vi "Cmd_G_OK.vi"(0 "Residence time":i32=100, 1 "PortNumber":i32=7, 2 "Command String":string) -> (3 "Received String1":string, 4 "Received String2":string, 5 "Received String3":string, 6 "OK Done":bool)   [LabVIEW 2015]
panel:
  # "Port Number 0=COM1"
  # "Send 'Command String', receive 'OK', send 'G Command' and receive 'OK'."
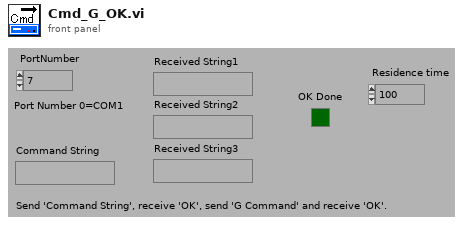
[diagram p1: front panel]
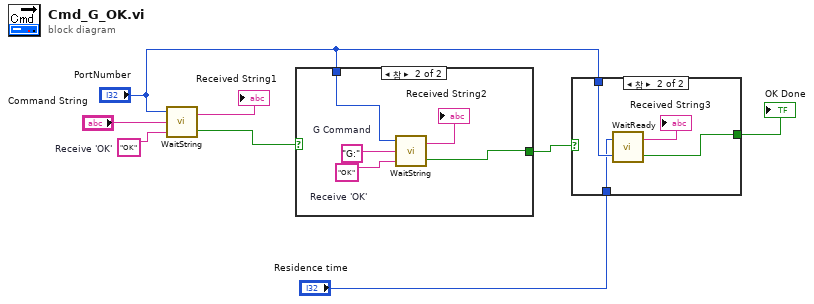
[diagram p0: block diagram]
diagram:
  w4 = "OK"  # Receive 'OK'
  n1 = call "WaitString.vi"("String to Receive"=w4, "String to Send"="Command String", "PortNumber"="PortNumber") -> ("OK Done"=w2:bool, "String Received"=→"Received String1":string)
  n2 = case shown="참" w2 {
    selector: w2 -> [w9 _]
    tunnel: "PortNumber" -> [_ w14]
    tunnel: [w9 w10] -> w7
    frame False {
    }
    frame True {
      w12 = "OK"  # Receive 'OK'
      w13 = "G:"  # G Command
      n3 = call "WaitString.vi"("String to Receive"=w12, "String to Send"=w13, "PortNumber"=w14) -> ("OK Done"=w10:bool, "String Received"=→"Received String2":string)
    }
  }
  n4 = case shown="참" w7 {
    selector: w7 -> [w15 _]
    tunnel: "PortNumber" -> [_ w19]
    tunnel: [w15 w17] -> w8
    tunnel: "Residence time" -> [_ w16]
    frame False {
    }
    frame True {
      n5 = call "WaitReady.vi"("PortNumber"=w19, "Residence time in ms"=w16) -> ("OK Done"=w17:bool, "String Received"=→"Received String3":string)
    }
  }
  "OK Done" <- w8
